vi "Get VISA User Data.vi"(8 "error in (no error)":errorcluster, 11 "VISA Refnum in":refnum<visa-resource-name>) -> (0 "error out":errorcluster, 2 "User Data":i32, 3 "VISA Refnum out":refnum<visa-resource-name>)   [LabVIEW 2019, in "KH7008.lvlib"]
uses:
  KH7008.lvlib
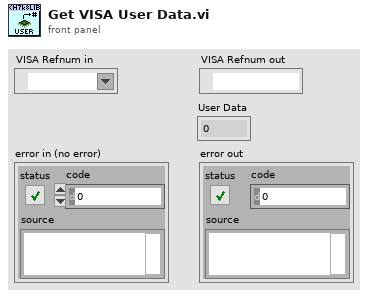
[diagram p1: front panel]
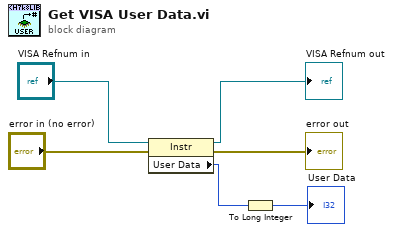
[diagram p0: block diagram]
diagram:
  n1 = property class="Instr"(reference="VISA Refnum in", error in="error in (no error)") -> (reference out=→"VISA Refnum out":refnum<visa-resource-name>, error out=→"error out":errorcluster, "User Data"=w2:u32)
  n2 = To Long Integer(number=w2) -> (32bit integer=→"User Data":i32)
